vi "题目1.vi"() -> ()   [LabVIEW 2017]
panel:
  out "添加的数组":dbl[](array[numeric])
  out "元素 4":dbl
  out "元素 3":dbl
  out "元素 2":dbl
  out "元素1":dbl
  out "数组":dbl[](array[numeric])
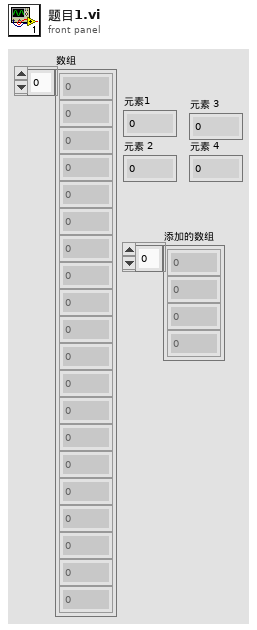
[diagram p1: front panel]
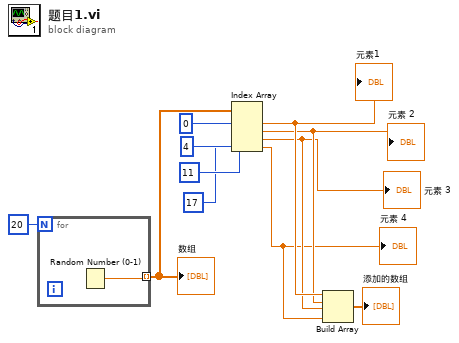
[diagram p0: block diagram]
diagram:
  n1 = for {
    N: 20 -> [_]
    tunnel: [w12] -> w11 mode=indexing
    n2 = Random Number (0-1)() -> (number: 0 to 1=w12:dbl)
  }
  "数组" <- w11
  n3 = Index Array(array=w11, index #1=0 ("索引"), index #2=4 ("索引"), index #3=11 ("索引"), index #4=17 ("索引")) -> (element #1=w6:dbl, element #2=w5:dbl, element #3=w4:dbl, element #4=w3:dbl)
  "元素1" <- w6
  "元素 2" <- w5
  "元素 3" <- w4
  "元素 4" <- w3
  n4 = Build Array(w6, w5, w4, w3) -> (→"添加的数组":dbl[])
